vi "week05_Ex01.vi"() -> ()   [LabVIEW 2017]
panel:
  out "Y":i32[](array[numeric])
  out "X":i32
  in  "stop 2":bool
  out "While round":i32
  out "Fol round":i32
  in  "stop":bool
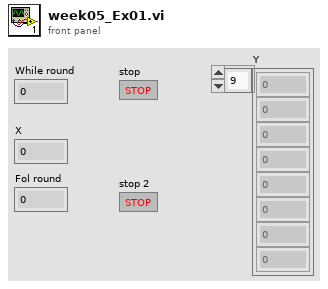
[diagram p1: front panel]
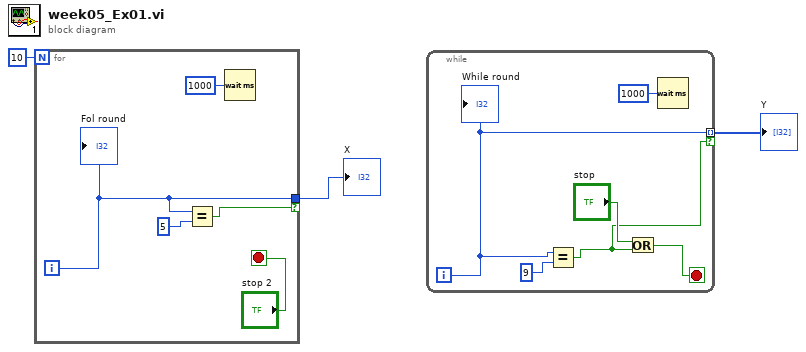
[diagram p0: block diagram]
diagram:
  n1 = for {
    N: 10 -> [_]
    tunnel: [w6] -> w2 if=w4
    i -> [w6]
    stop <- "stop 2" stop-if-true
    n2 = Equal?(x=w6, y=5) -> (x = y?=w4:bool)
    n3 = Wait (ms)(milliseconds to wait=u32 1000) -> ()  [unwired: 1 out]
    "Fol round" <- w6
  }
  "X" <- w2
  n4 = while {
    tunnel: [w10] -> w1 mode=indexing if=w9
    i -> [w10]
    stop <- w11 stop-if-true
    n5 = Equal?(x=w10, y=9) -> (x = y?=w9:bool)
    n6 = Or(x="stop", y=w9) -> (x .or. y?=w11:bool)
    n7 = Wait (ms)(milliseconds to wait=u32 1000) -> ()  [unwired: 1 out]
    "While round" <- w10
  }
  "Y" <- w1
